vi "curve.vi"(2 "error out 4":errorcluster, 3 "VISA resource name 4":refnum<visa-resource-name>) -> (0 "error out 5":errorcluster, 1 "VISA resource name 5":refnum<visa-resource-name>)   [LabVIEW 2017]
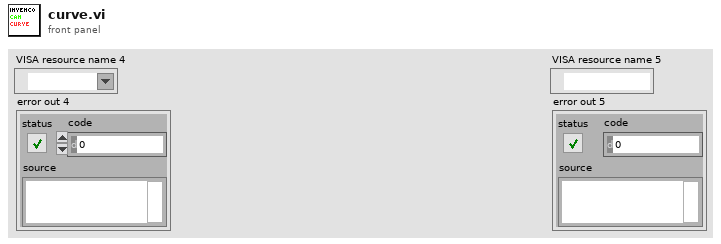
[diagram p1: front panel]
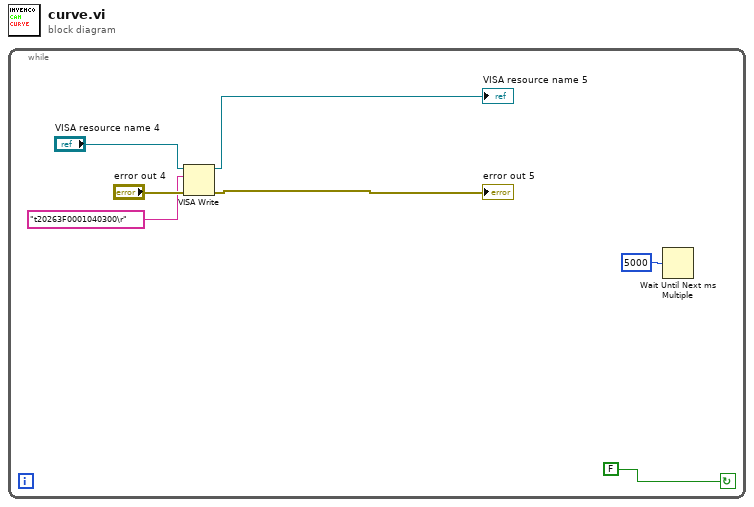
[diagram p0: block diagram]
diagram:
  n1 = while {
    stop <- FALSE continue-if-true
    n2 = VISA Write(VISA resource name="VISA resource name 4", write buffer="t20263F0001040300\r", error in (no error)="error out 4") -> (VISA resource name out=→"VISA resource name 5":refnum<visa-resource-name>, error out=→"error out 5":errorcluster)  [unwired: 1 out]
    n3 = Wait Until Next ms Multiple(millisecond multiple=u32 5000) -> ()  [unwired: 1 out]
  }
